vi "Get Object from Test.vi"(11 "Executioner in":refnum<class "Executioner.lvclass">) -> (1 "Test":refnum<class>, 3 "Executioner out":refnum<class "Executioner.lvclass">)   [LabVIEW 2017, in "Test Executive.lvlib" / "Executioner.lvclass"]
uses:
  <vilib>/gpm_packages/@cs/test-executive/Source/Test Executive/Executioner/Executioner.lvclass
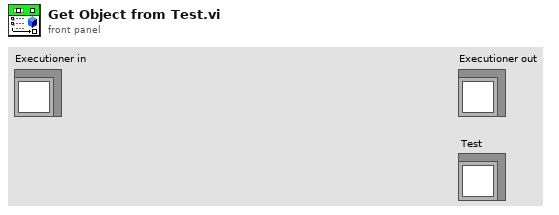
[diagram p1: front panel]
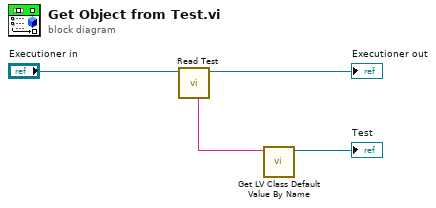
[diagram p0: block diagram]
diagram:
  n1 = call <vilib>:"Read Test.vi"("Executioner in"="Executioner in") -> ("Executioner out"=→"Executioner out":refnum<class "Executioner.lvclass">, "Test"=w2:string)  [unwired: 9 in]
  n2 = call <vilib>:"Get LV Class Default Value By Name.vi"("class name"=w2) -> ("object"=→"Test":refnum<class>)  [unwired: 9 in, 1 out]
